vi "de6face.vi"() -> ()   [LabVIEW 2018]
panel:
  in  "Numéro":dbl=1.0 min=1.0 max=6.0 step=1.0
  out "7":bool
  out "6":bool
  out "3":bool
  out "5":bool
  out "2":bool
  out "4":bool
  out "1":bool
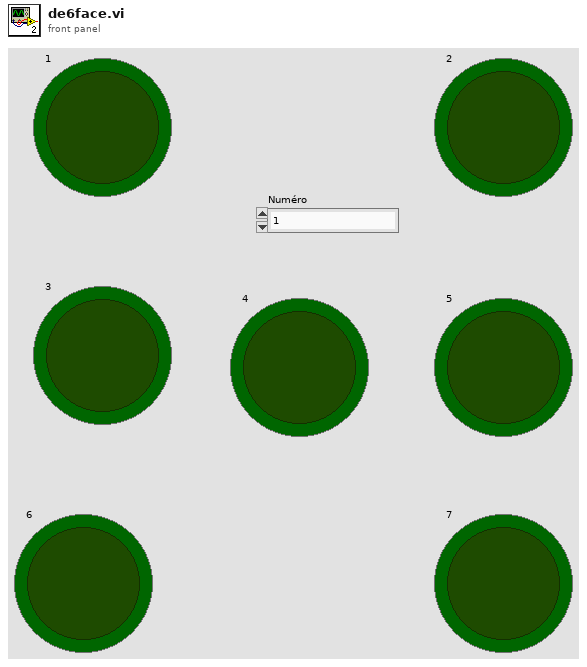
[diagram p1: front panel]
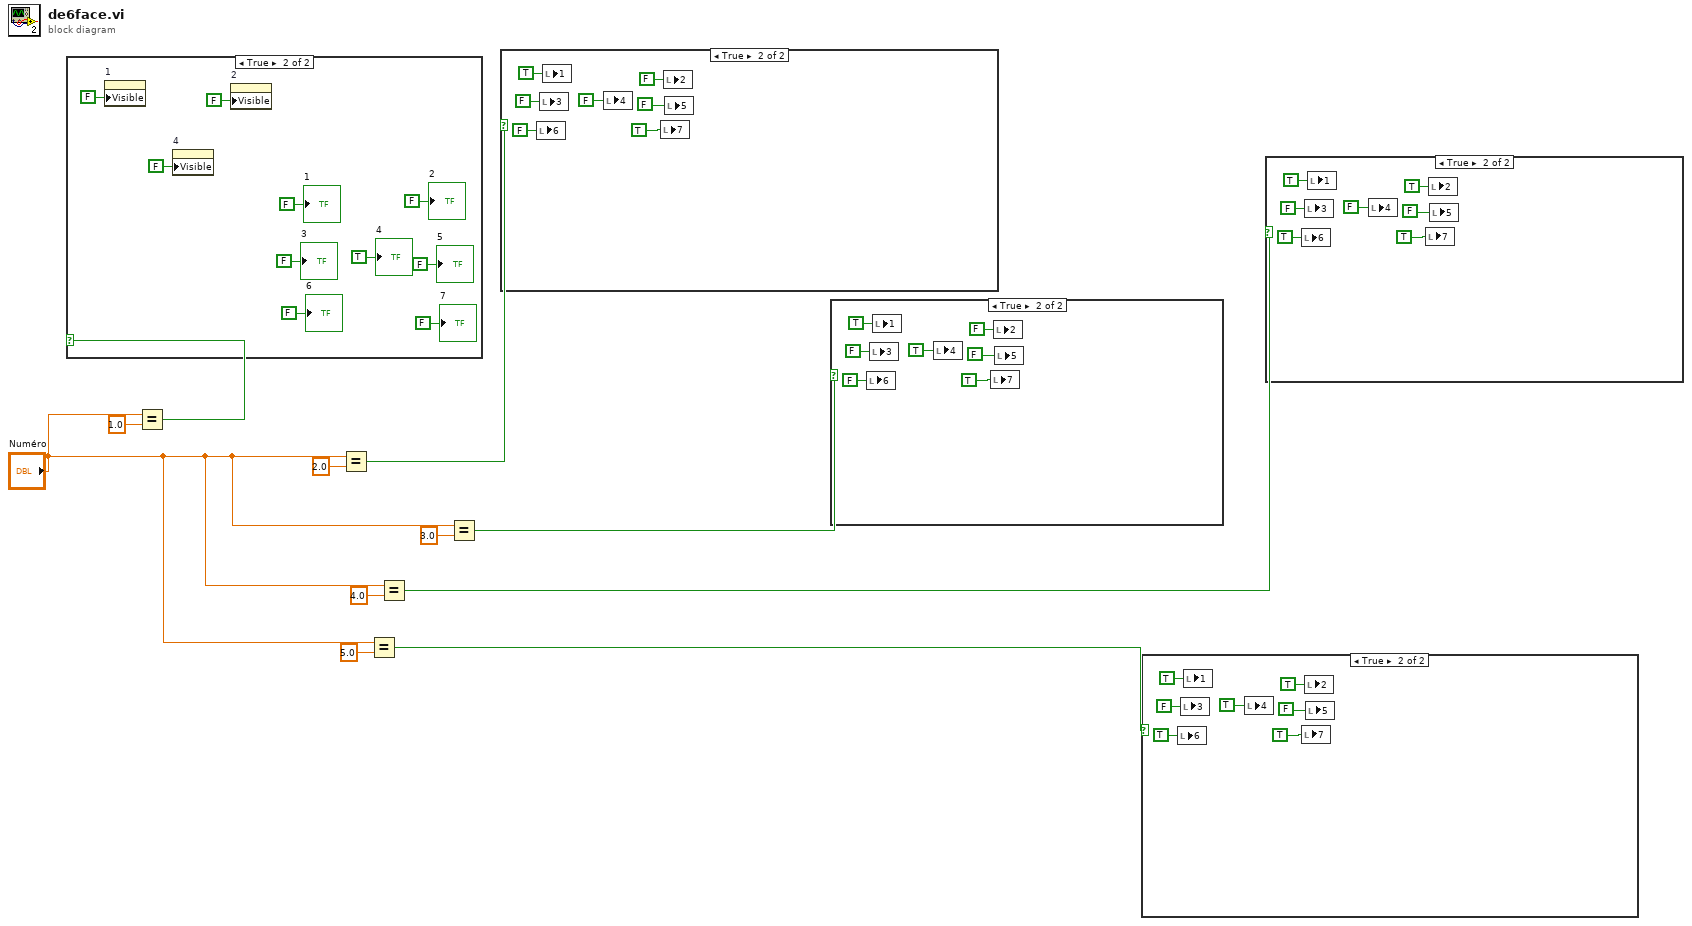
[diagram p0: block diagram]
diagram:
  n1 = Equal?(x="Numéro", y=1.0) -> (x = y?=w11:bool)
  n2 = case shown="True" w11 {
    frame False {
    }
    frame True {
      n3 = property on="1" class="Bool (strict)"("Visible"=FALSE) -> ()  [unwired: 2 in, 2 out]
      n4 = property on="4" class="Bool (strict)"("Visible"=FALSE) -> ()  [unwired: 2 in, 2 out]
      n5 = property on="2" class="Bool (strict)"("Visible"=FALSE) -> ()  [unwired: 2 in, 2 out]
      "1" <- FALSE
      "4" <- TRUE
      "2" <- FALSE
      "5" <- FALSE
      "3" <- FALSE
      "6" <- FALSE
      "7" <- FALSE
    }
  }
  n6 = Equal?(x="Numéro", y=2.0) -> (x = y?=w8:bool)
  n7 = Equal?(x="Numéro", y=5.0) -> (x = y?=w1:bool)
  n8 = Equal?(x="Numéro", y=4.0) -> (x = y?=w2:bool)
  n9 = Equal?(x="Numéro", y=3.0) -> (x = y?=w3:bool)
  n10 = case shown="True" w8 {
    frame False {
    }
    frame True {
      n11 = local write "6"(FALSE ("1")) -> ()
      n12 = local write "3"(FALSE ("1")) -> ()
      n13 = local write "1"(TRUE ("1")) -> ()
      n14 = local write "4"(FALSE ("1")) -> ()
      n15 = local write "7"(TRUE ("1")) -> ()
      n16 = local write "2"(FALSE ("1")) -> ()
      n17 = local write "5"(FALSE ("1")) -> ()
    }
  }
  n18 = case shown="True" w3 {
    frame False {
    }
    frame True {
      n19 = local write "6"(FALSE ("1")) -> ()
      n20 = local write "3"(FALSE ("1")) -> ()
      n21 = local write "1"(TRUE ("1")) -> ()
      n22 = local write "4"(TRUE ("1")) -> ()
      n23 = local write "7"(TRUE ("1")) -> ()
      n24 = local write "2"(FALSE ("1")) -> ()
      n25 = local write "5"(FALSE ("1")) -> ()
    }
  }
  n26 = case shown="True" w1 {
    frame False {
    }
    frame True {
      n27 = local write "6"(TRUE ("1")) -> ()
      n28 = local write "3"(FALSE ("1")) -> ()
      n29 = local write "1"(TRUE ("1")) -> ()
      n30 = local write "4"(TRUE ("1")) -> ()
      n31 = local write "7"(TRUE ("1")) -> ()
      n32 = local write "2"(TRUE ("1")) -> ()
      n33 = local write "5"(FALSE ("1")) -> ()
    }
  }
  n34 = case shown="True" w2 {
    frame False {
    }
    frame True {
      n35 = local write "6"(TRUE ("1")) -> ()
      n36 = local write "3"(FALSE ("1")) -> ()
      n37 = local write "1"(TRUE ("1")) -> ()
      n38 = local write "4"(FALSE ("1")) -> ()
      n39 = local write "7"(TRUE ("1")) -> ()
      n40 = local write "2"(TRUE ("1")) -> ()
      n41 = local write "5"(FALSE ("1")) -> ()
    }
  }
